vi "Read Flipped.vi"(9 "Scale in":refnum<class "Scale.lvclass">) -> (3 "Scale out":refnum<class "Scale.lvclass">, 4 "Flipped":bool)   [LabVIEW 2014, in "Scale.lvclass"]
uses:
  Scale.lvclass
  Scale.lvclass/Scale.ctl
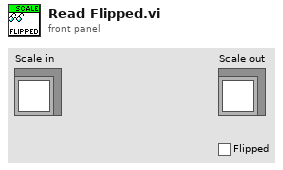
[diagram p1: front panel]
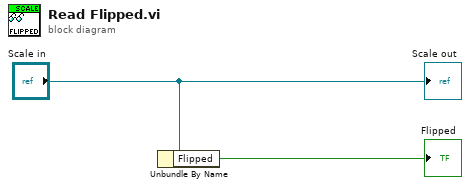
[diagram p0: block diagram]
diagram:
  n1 = Unbundle By Name("Scale in") -> ("Flipped"=→"Flipped":bool)
  "Scale out" <- "Scale in"
